vi "PH_Beckhoff_StepMot.Test.vi"() -> ()   [LabVIEW 2014, in "PH_Beckhoff_StepMot.lvlib"]
uses:
  PH_Beckhoff_StepMot.lvlib
  PH_Stepmotor_BaseClass/PH_Stepmotor_BaseClass.Axis Activity.ctl
  non_GPL/instr.lib/Beckhoff/Read and Write Data/Step Motor Klemmen/Beckhoff.Step Motor - Control Byte.ctl
  non_GPL/instr.lib/Beckhoff/Read and Write Data/Step Motor Klemmen/Beckhoff.Step Motor - Control Word.ctl
  non_GPL/instr.lib/Beckhoff/Specials/Step Motor Klemmen/Beckhoff.Step Motor - Motor Configuration.ctl
  non_GPL/instr.lib/Beckhoff/Read and Write Register/Step Motor Klemmen/Beckhoff.Step Motor - Feature Register 1.ctl
  non_GPL/instr.lib/Beckhoff/Read and Write Register/Step Motor Klemmen/Beckhoff.Step Motor - Feature Register 2.ctl
  non_GPL/instr.lib/Beckhoff/Specials/Step Motor Klemmen/Beckhoff.Step Motor - Klemmen.ctl
  non_GPL/instr.lib/Beckhoff/Read and Write Data/Step Motor Klemmen/Beckhoff.Step Motor - Status.ctl
  non_GPL/instr.lib/Beckhoff/Read and Write Data/Step Motor Klemmen/Beckhoff.Step Motor - Status Byte.ctl
  non_GPL/instr.lib/Beckhoff/Read and Write Data/Step Motor Klemmen/Beckhoff.Step Motor - Status Word.ctl
  non_GPL/instr.lib/Beckhoff/Helpers/Beckhoff Access.ctl
  non_GPL/instr.lib/Beckhoff/Helpers/Klemmendeclarer.ctl
  non_GPL/instr.lib/Beckhoff/Beckhoff - Driver np.lvlib
  PH_Common/PH_Common.lvlib
  PH_Stepmotor_BaseClass/PH_Stepmotor_BaseClass.lvlib
panel:
  in  "Go to":bool
  in  "goto pos":i32
  out "Status":T1
  out "Klemmentype":T4
  out "Position":cluster{"Target":i32, "Current":i32}
  in  "Tab Control":T5(tab)
  in  "Configuration":T6
  in  "ES enabled":bool
  in  "ES reversed":bool caption="End-Switches reversed"
  in  "Set Position":bool
  in  "Position to set":i32=10000
  in  "Register Value to set":u32 caption="Value to set"
  in  "Set Register":bool caption="Set Register Word"
  in  "Register":u32
  in  "Read Register":bool caption="Read"
  out "Register Current Value":u32 caption="Current Value"
  in  "Set Control Word":bool caption="Set Word"
  in  "Set Control Byte":bool caption="Set Byte"
  in  "Control Word":T9 caption="Word"
  in  "Control Byte":T10 caption="Byte"
  in  "Set Dig Outs":bool[](array[boolean])
  out "Current Dig Outs":bool[](array[boolean])
  out "Current Dig Ins":bool[](array[boolean])
  out "Config ready":bool
  out "Coupler found":bool
  out "Client found":bool
  out "Successfully pinged?":bool
  in  "IP":string="192.168.0.231"
  out "Error Code":string
  out "DLL Error":errorcluster
  out "Port opened?":bool
  out "Close successful":bool
  in  "Stop":bool
  out "Axis Activity":T11=enum."stopped"
  out "Loop Counter":i32
  in  "End":bool
  in  "Reset Klemme":bool
  in  "Klemme":u32=2
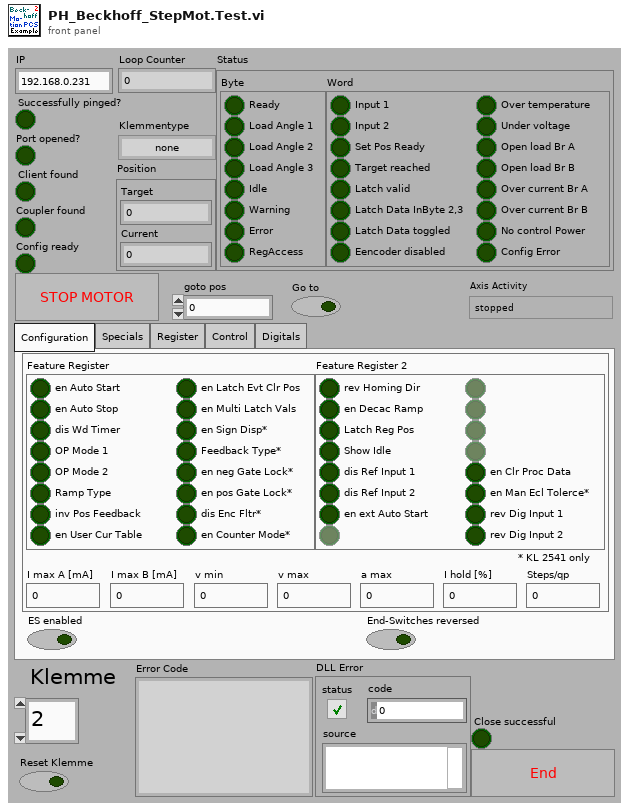
[diagram p1: front panel]
types:
  T1 = typedef "Beckhoff - Driver np.lvlib/Beckhoff.Step Motor - Status.ctl" = cluster{"Byte":T2, "Word":T3}
  T2 = typedef "Beckhoff - Driver np.lvlib/Beckhoff.Step Motor - Status Byte.ctl" = cluster{"Ready":bool, "Load Angle 1":bool, "Load Angle 2":bool, "Load Angle 3":bool, "Idle":bool, "Warning":bool, "Error":bool, "RegAccess":bool}
  T3 = typedef "Beckhoff - Driver np.lvlib/Beckhoff.Step Motor - Status Word.ctl" = cluster{"Input 1":bool, "Input 2":bool, "Set Pos Ready":bool, "Target reached":bool, "Latch valid":bool, "Latch Data InByte 2,3":bool, "Latch Data toggled":bool, "Eencoder disabled":bool, "Over temperature":bool, "Under voltage":bool, "Open load Br A":bool, "Open load Br B":bool, "Over current Br A":bool, "Over current Br B":bool, "No control Power":bool, "Config Error":bool}
  T4 = typedef "Beckhoff - Driver np.lvlib/Beckhoff.Step Motor - Klemmen.ctl" = enum16{"none", "KL 2531", "KL 2541"}
  T5 = enum32{"Configuration", "Specials", "Register", "Control", "Digitals"}
  T6 = typedef "Beckhoff - Driver np.lvlib/Beckhoff.Step Motor - Motor Configuration.ctl" = cluster{"Feature Register":T7, "I max A [mA]":dbl, "I max B [mA]":dbl, "v min":u32, "v max":u32, "a max":u32, "I hold [%]":u32, "Steps/qp":u32, "Feature Register 2":T8}
  T7 = typedef "Beckhoff - Driver np.lvlib/Beckhoff.Step Motor - Feature Register 1.ctl" = cluster{"en Auto Start":bool, "en Auto Stop":bool, "dis Wd Timer":bool, "OP Mode 1":bool, "OP Mode 2":bool, "Ramp Type":bool, "inv Pos Feedback":bool, "en User Cur Table":bool, "en Latch Evt Clr Pos":bool, "en Multi Latch Vals":bool, "en Sign Disp*":bool, "Feedback Type*":bool, "en neg Gate Lock*":bool, "en pos Gate Lock*":bool, "dis Enc Fltr*":bool, "en Counter Mode*":bool}
  T8 = typedef "Beckhoff - Driver np.lvlib/Beckhoff.Step Motor - Feature Register 2.ctl" = cluster{"rev Homing Dir":bool, "en Decac Ramp":bool, "Latch Reg Pos":bool, "Show Idle":bool, "dis Ref Input 1":bool, "dis Ref Input 2":bool, "en ext Auto Start":bool, "N/A":bool, "N/A":bool, "N/A":bool, "N/A":bool, "N/A":bool, "en Clr Proc Data":bool, "en Man Ecl Tolerce*":bool, "rev Dig Input 1":bool, "rev Dig Input 2":bool}
  T9 = typedef "Beckhoff - Driver np.lvlib/Beckhoff.Step Motor - Control Word.ctl" = cluster{"en Latch C":bool, "en Latch Input 1":bool, "en Latch Input 2":bool, "en Latch Rise Edge":bool, "en Latch Fall Edge":bool, "Get Latch Data":bool, "Toggle Latch Data":bool, "Get Position Error":bool, "Get Encoder Position":bool, "Dis mixed Decay":bool, "Set Pos":bool, "Reduced Current":bool, "Reduced Current (drivng)":bool, "Clear Position":bool, "Set Position in Process Data":bool, "N/A":bool}
  T10 = typedef "Beckhoff - Driver np.lvlib/Beckhoff.Step Motor - Control Byte.ctl" = cluster{"Enable":bool, "PLC-Stop":bool, "Start":bool, "Red Current":bool, "AutoStart":bool, "AutoStop":bool, "Reset":bool, "RegAccess":bool}
  T11 = typedef "PH_Stepmotor_BaseClass.lvlib/PH_Stepmotor_BaseClass.Axis Activity.ctl" = enum16{"No Information", "stopped", "running", "Failure", "Alarm", "stopped at backward ES", "stopped at foreward ES"}
  T12 = typedef "Beckhoff - Driver np.lvlib/Klemmendeclarer.ctl" = cluster{"Offset due to Sonderklemms":u32, "analog Inputs":u32, "analog Outputs":u32, "digital Input Bits":u32, "digital Output Bits":u32}
  T13 = typedef "Beckhoff - Driver np.lvlib/Beckhoff Access.ctl" = cluster{"DLL path":path, "AMS Net ID":cluster{"1st # of IP":u8, "2nd # of IP":u8, "3rd # of IP":u8, "4th # of IP":u8, "In Port":u8, "Out Port":u8}}
  T14 = cluster{"1st # of IP":u8, "2nd # of IP":u8, "3rd # of IP":u8, "4th # of IP":u8, u8, u8}
  T15 = enum8{"Enabled", "Disabled", "Disabled and Grayed Out"}
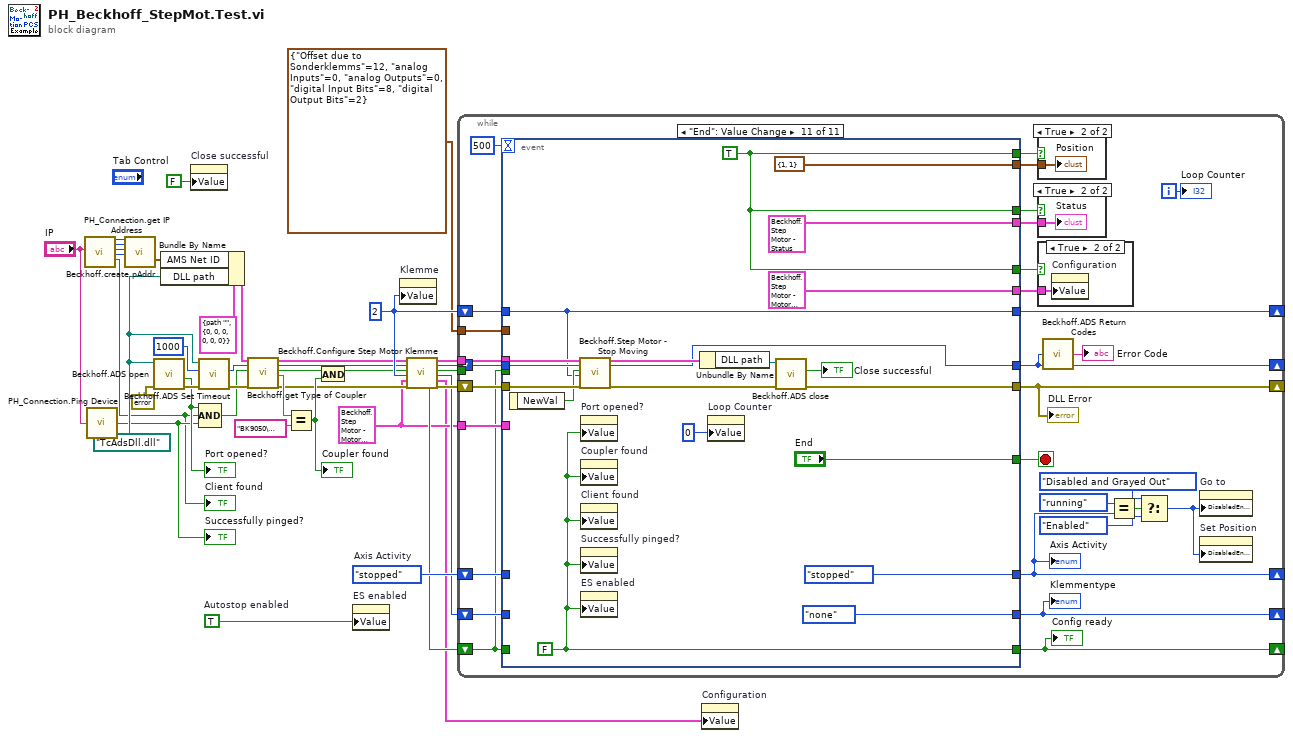
[diagram p0: block diagram]
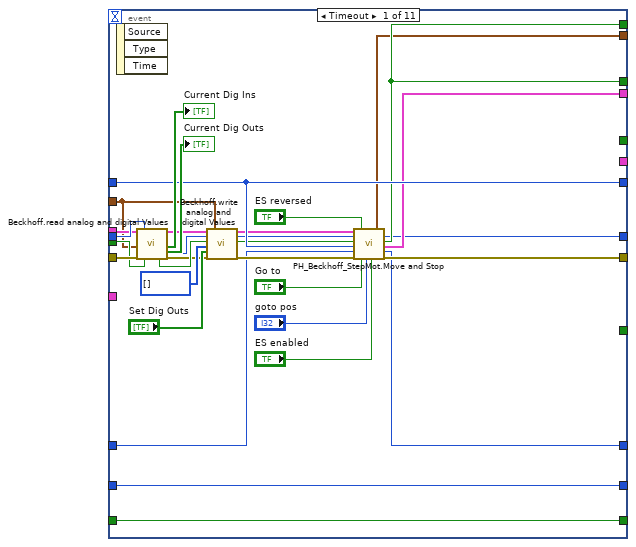
[diagram p5: hidden frame]
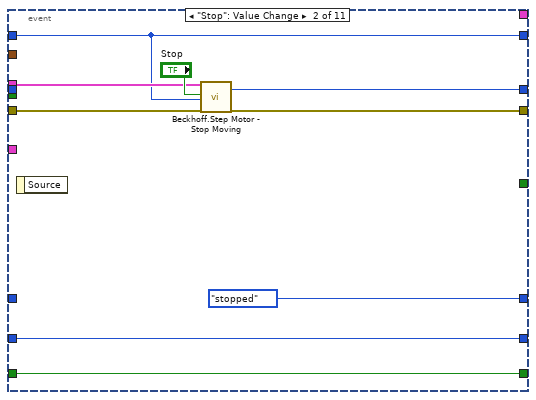
[diagram p6: hidden frame]
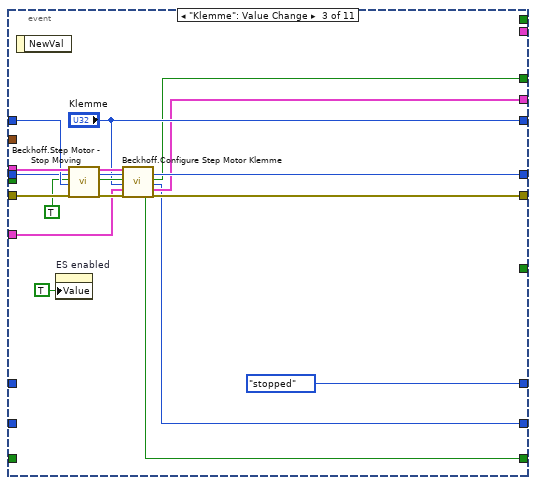
[diagram p7: hidden frame]
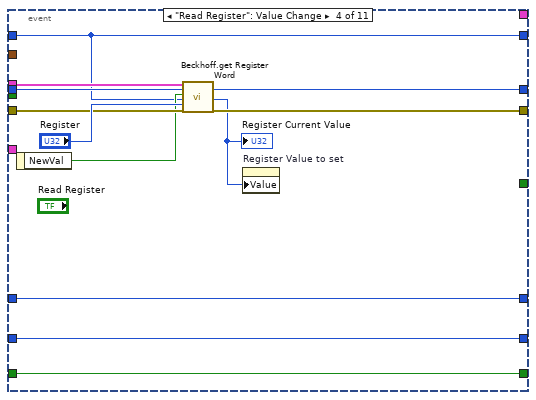
[diagram p8: hidden frame]
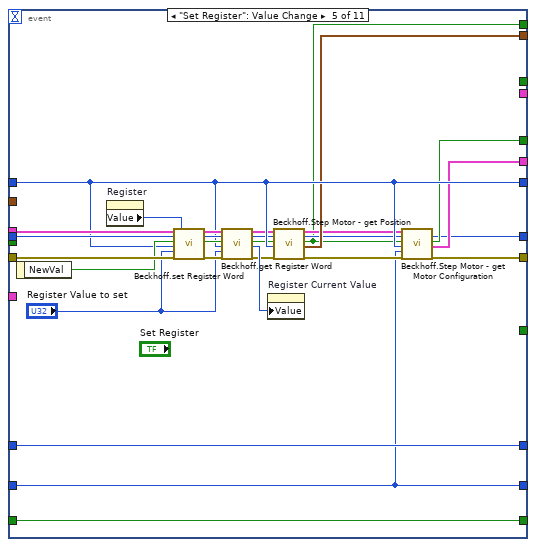
[diagram p9: hidden frame]
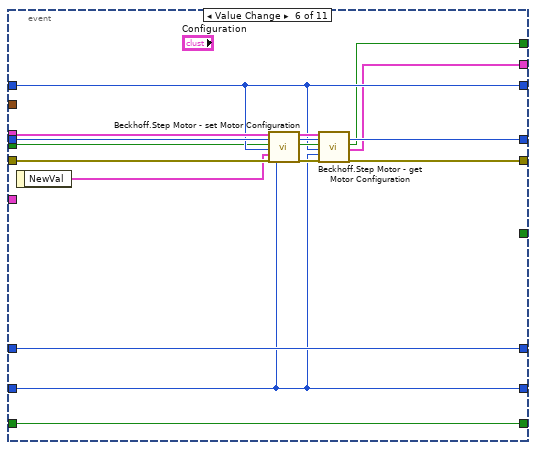
[diagram p10: hidden frame]
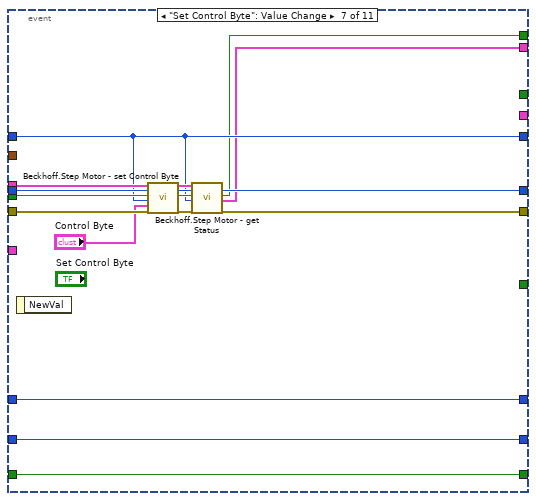
[diagram p11: hidden frame]
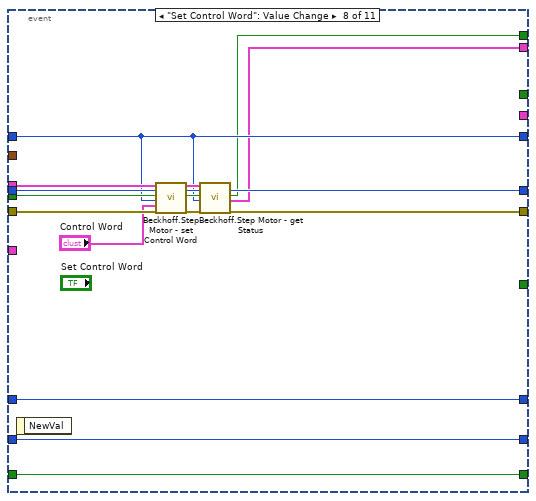
[diagram p12: hidden frame]
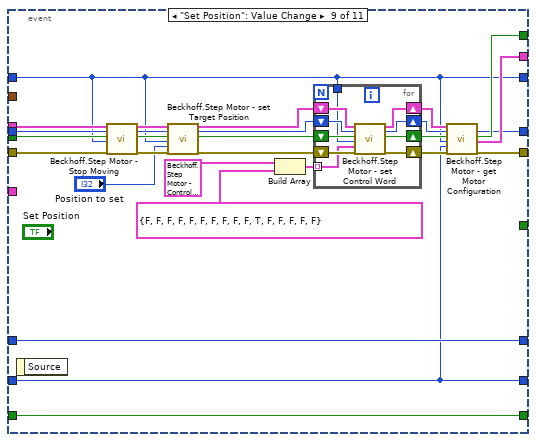
[diagram p13: hidden frame]
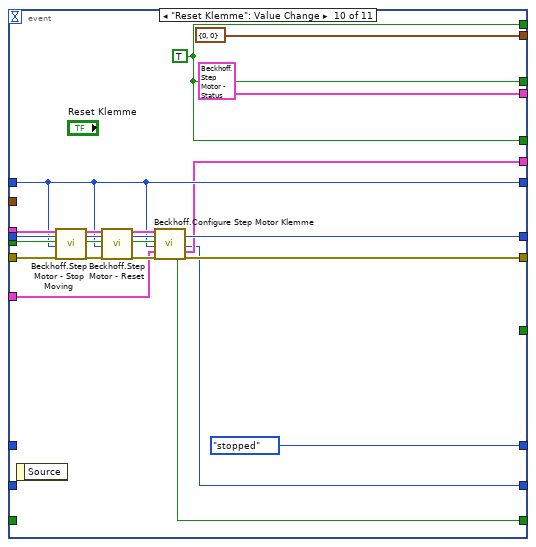
[diagram p14: hidden frame]
diagram:
  w2 = T6 {"Feature Register"={"en Auto Start"=FALSE, "en Auto Stop"=TRUE, "dis Wd Timer"=TRUE, "OP Mode 1"=TRUE, "OP Mode 2"=TRUE, "Ramp Type"=FALSE, "inv Pos Feedback"=FALSE, "en User Cur Table"=FALSE, "en Latch Evt Clr Pos"=FALSE, "en Multi Latch Vals"=FALSE, "en Sign Disp*"=FALSE, "Feedback Type*"=FALSE, "en neg Gate Lock*"=FALSE, "en pos Gate Lock*"=FALSE, "dis Enc Fltr*"=FALSE, "en Counter Mode*"=FALSE}, "I max A [mA]"=400.0, "I max B [mA]"=400.0, "v min"=10, "v max"=512, "a max"=32, "I hold [%]"=15, "Steps/qp"=4, "Feature Register 2"={"rev Homing Dir"=FALSE, "en Decac Ramp"=FALSE, "Latch Reg Pos"=FALSE, "Show Idle"=TRUE, "dis Ref Input 1"=FALSE, "dis Ref Input 2"=FALSE, "en ext Auto Start"=FALSE, "N/A"=FALSE, "N/A"=FALSE, "N/A"=FALSE, "N/A"=FALSE, "N/A"=FALSE, "en Clr Proc Data"=FALSE, "en Man Ecl Tolerce*"=FALSE, "rev Dig Input 1"=TRUE, "rev Dig Input 2"=TRUE}} ("Micos VT-80")
  w12 = u32 2 ("Klemme")
  w15 = TRUE  # Autostop enabled
  w16 = PH_Stepmotor_BaseClass.Axis_Activity."stopped"  # Axis Activity
  w31 = path "TcAdsDll.dll" ("DLL path in")
  n1 = call "PH_Connection.get IP Address.vi"("IP Name"="IP") -> ("1st # of IP"=w39:u8, "2nd # of IP"=w38:u8, "3rd # of IP"=w37:u8, "4th # of IP"=w36:u8, "Client found"=w19:bool)  [unwired: 13 in, 1 out]
  "Client found" <- w19
  n2 = call "PH_Connection.Ping Device.vi"("IP"="IP") -> ("successfully pinged?"=w25:bool)
  "Successfully pinged?" <- w25
  n3 = call "Beckhoff.create pAddr.vi"("1st # of IP"=w39, "2nd # of IP"=w38, "3rd # of IP"=w37, "4th # of IP"=w36) -> ("AMS Net ID"=w21:T14)  [unwired: 13 in, 2 out]
  n4 = call "Beckhoff.ADS open.vi"("error in"=errorcluster {"status"=FALSE, "code"=0, "source"=""}, "path in"=w31) -> ("error out"=w33:errorcluster, "Port opened?"=w26:bool)  [unwired: 3 in, 1 out]
  "Port opened?" <- w26
  n5 = Bundle By Name(cluster=T13 {"DLL path"=path "", "AMS Net ID"={"1st # of IP"=0, "2nd # of IP"=0, "3rd # of IP"=0, "4th # of IP"=0, "In Port"=0, "Out Port"=0}} ("AMS Net ID in"), "AMS Net ID"=w21, "DLL path"=w31) -> (w29:T13)
  n6 = property on="Close successful" class="Bool (strict)"("Value"=FALSE ("coupler found")) -> ()  [unwired: 2 in, 2 out]
  n7 = call "Beckhoff.ADS Set Timeout.vi"("error in"=w33, "nMs in"=u32 1000 ("nMs"), "path in"=w31) -> ("error out"=w27:errorcluster, "return type"=w28:i32)  [unwired: 6 in, 1 out]
  n8 = Compound Arithmetic op=AND(w26, w19, w25) -> (w24:bool)
  n9 = call "Beckhoff.get Type of Coupler.vi"("AMS Net ID in"=w29, "ADS Error in (0)"=w28, "Read?"=w24, "error in"=w27) -> ("AMS Net ID out"=w11:T13, "ADS Error out"=w10:i32, "Read successful?"=w17:bool, "Coupler Type"=w22:string, "error out"=w14:errorcluster)  [unwired: 11 in]
  n10 = Equal?(x=w22, y="BK9050\u0000\u0000" ("type")) -> (x = y?=w18:bool)
  "Coupler found" <- w18
  n11 = And(x=w17, y=w18) -> (x .and. y?=w9:bool)
  n12 = property on="ES enabled" class="Bool (strict)"("Value"=w15) -> ()  [unwired: 2 in, 2 out]
  n13 = property on="Klemme" class="DigNum (strict)"("Value"=w12) -> ()  [unwired: 2 in, 2 out]
  n14 = call "Beckhoff.Configure Step Motor Klemme.vi"("AMS Net ID in"=w11, "ADS Error in"=w10, "Configure?"=w9, "Klemme"=w12, "Default Configuration"=w2, "error in (no error)"=w14) -> ("Successfully configured?"=w4:bool, "AMS Net ID out"=w8:T13, "ADS Error out"=w7:i32, "Operation successful?"=w6:bool, "Klemmentype"=w5:T4, "Current Step Motor Configuration"=w1:T6, "error out"=w13:errorcluster)  [unwired: 7 in]
  n15 = while {
    shift-right: [w42] -> _
    shift-left: w16 -> [w68]
    tunnel: w8 -> [w67]
    tunnel: w6 -> [_]
    shift-right: [w61] -> _
    shift-left: w13 -> [w65]
    shift-right: [w60] -> _
    shift-left: w7 -> [w64]
    shift-right: [w57] -> _
    shift-left: w12 -> [w66]
    shift-right: [w49] -> _
    shift-left: w5 -> [w58]
    tunnel: w2 -> [w52]
    shift-right: [w48] -> _
    shift-left: w4 -> [w47]
    tunnel: T12 {"Offset due to Sonderklemms"=12, "analog Inputs"=0, "analog Outputs"=0, "digital Input Bits"=8, "digital Output Bits"=2} ("Klemmendeclarer: # of") -> [w43]
    i -> [w69]
    stop <- w62 stop-if-true
    n16 = event shown="[10] \"End\": Value Change" {
      selector: _ -> [_ _ _ _ _ _ _ _ _ _ _]
      dyn-events: _ -> [_ _ _ _ _ _ _ _ _ _ _]
      timeout: 500 -> [_ _ _ _ _ _ _ _ _ _ _]
      tunnel: w68 -> [w76 _ _ w141 w171 w188 w190 w207 w235 _ _]
      tunnel: [w86 PH_Stepmotor_BaseClass.Axis_Activity."stopped" ("Moving: 0: No; 1: forward; -1: backward") PH_Stepmotor_BaseClass.Axis_Activity."stopped" ("Moving: 0: No; 1: forward; -1: backward") w141 w171 w188 w190 w207 w235 PH_Stepmotor_BaseClass.Axis_Activity."stopped" ("Moving: 0: No; 1: forward; -1: backward") PH_Stepmotor_BaseClass.Axis_Activity."stopped" ("Moving: 0: No; 1: forward; -1: backward")] -> w42
      tunnel: w67 -> [w90 w109 w131 w139 w170 w187 w205 w222 w243 w283 w300]
      tunnel: w66 -> [w85 w107 w129 w134 w159 w177 w194 w211 w224 w268 w292]
      tunnel: w47 -> [w92 _ _ _ _ w172 w202 w219 w241 w281 _]
      tunnel: [w87 w111 w117 w143 w146 w180 w196 w214 w234 w266 w294] -> w61
      tunnel: w65 -> [w93 w108 w130 w137 w168 w185 w204 w221 w240 w280 w298]
      tunnel: [w80 w112 w125 w142 w147 w179 w195 w213 w227 w265 w293] -> w60
      tunnel: w64 -> [w91 _ w127 w138 w169 w186 w203 w220 w242 w282 w295]
      tunnel: [_ _ _ _ _ _ _ _ _ _ "End"] -> w62
      tunnel: w58 -> [w102 w106 _ w133 w145 w176 w191 w208 w225 _ _]
      tunnel: [w85 w107 "Klemme" w134 w159 w177 w194 w211 w224 w268 w292] -> w57
      tunnel: [w83 _ _ _ w150 _ _ _ _ w273 w289] -> w56
      tunnel: [w82 _ _ _ w158 _ _ _ _ cluster{"Target":i32, "Current":i32} {"Target"=0, "Current"=0} ("Position 2") cluster{"Target":i32, "Current":i32} {"Target"=1, "Current"=1} ("Position")] -> w55
      tunnel: [w83 _ _ _ _ _ w193 w209 _ w273 w289] -> w54
      tunnel: [w81 _ _ _ _ _ w192 w210 _ T1 {"Byte"={"Ready"=FALSE, "Load Angle 1"=FALSE, "Load Angle 2"=FALSE, "Load Angle 3"=FALSE, "Idle"=FALSE, "Warning"=FALSE, "Error"=FALSE, "RegAccess"=FALSE}, "Word"={"Input 1"=FALSE, "Input 2"=FALSE, "Set Pos Ready"=FALSE, "Target reached"=FALSE, "Latch valid"=FALSE, "Latch Data InByte 2,3"=FALSE, "Latch Data toggled"=FALSE, "Eencoder disabled"=FALSE, "Over temperature"=FALSE, "Under voltage"=FALSE, "Open load Br A"=FALSE, "Open load Br B"=FALSE, "Over current Br A"=FALSE, "Over current Br B"=FALSE, "No control Power"=FALSE, "Config Error"=FALSE}} ("Status") T1 {"Byte"={"Ready"=FALSE, "Load Angle 1"=FALSE, "Load Angle 2"=FALSE, "Load Angle 3"=FALSE, "Idle"=FALSE, "Warning"=FALSE, "Error"=FALSE, "RegAccess"=FALSE}, "Word"={"Input 1"=FALSE, "Input 2"=FALSE, "Set Pos Ready"=FALSE, "Target reached"=FALSE, "Latch valid"=FALSE, "Latch Data InByte 2,3"=FALSE, "Latch Data toggled"=FALSE, "Eencoder disabled"=FALSE, "Over temperature"=FALSE, "Under voltage"=FALSE, "Open load Br A"=FALSE, "Open load Br B"=FALSE, "Over current Br A"=FALSE, "Over current Br B"=FALSE, "No control Power"=FALSE, "Config Error"=FALSE}} ("Status")] -> w53
      tunnel: [_ _ w119 _ w148 w174 _ _ w228 w273 w289] -> w51
      tunnel: [_ _ w118 _ w157 w173 _ _ w229 w264 T6 {"Feature Register"={"en Auto Start"=FALSE, "en Auto Stop"=FALSE, "dis Wd Timer"=FALSE, "OP Mode 1"=FALSE, "OP Mode 2"=FALSE, "Ramp Type"=FALSE, "inv Pos Feedback"=FALSE, "en User Cur Table"=FALSE, "en Latch Evt Clr Pos"=FALSE, "en Multi Latch Vals"=FALSE, "en Sign Disp*"=FALSE, "Feedback Type*"=FALSE, "en neg Gate Lock*"=FALSE, "en pos Gate Lock*"=FALSE, "dis Enc Fltr*"=FALSE, "en Counter Mode*"=FALSE}, "I max A [mA]"=0.0, "I max B [mA]"=0.0, "v min"=0, "v max"=0, "a max"=0, "I hold [%]"=0, "Steps/qp"=0, "Feature Register 2"={"rev Homing Dir"=FALSE, "en Decac Ramp"=FALSE, "Latch Reg Pos"=FALSE, "Show Idle"=FALSE, "dis Ref Input 1"=FALSE, "dis Ref Input 2"=FALSE, "en ext Auto Start"=FALSE, "N/A"=FALSE, "N/A"=FALSE, "N/A"=FALSE, "N/A"=FALSE, "N/A"=FALSE, "en Clr Proc Data"=FALSE, "en Man Ecl Tolerce*"=FALSE, "rev Dig Input 1"=FALSE, "rev Dig Input 2"=FALSE}} ("Step Motor Configuration")] -> w50
      tunnel: [w102 w106 w115 w133 w145 w176 w191 w208 w225 w263 Beckhoff.Step_Motor_-_Klemmen."none" ("Klemmentype 2")] -> w49
      tunnel: w52 -> [_ _ w120 _ _ _ _ _ _ w267 _]
      tunnel: [w103 w105 w116 w132 w144 w175 w189 w206 w226 w262 w285] -> w48
      tunnel: w47 -> [w103 w105 _ w132 w144 w175 w189 w206 w226 _ _]
      tunnel: w43 -> [w89 _ _ _ _ _ _ _ _ _ _]
      event Timeout {
        n17 = event-data() -> ()  [unwired: 1 in, 3 out]
        n18 = call "Beckhoff.read analog and digital Values.vi"("AMS Net ID in"=w90, "Klemmendeclarer: # of"=w89, "error in"=w93, "ADS Error in (0)"=w91, "Read?"=w92) -> ("ADS Error out"=w97:i32, "read successful?"=w96:bool, "AMS Net ID out"=w94:T13, "Current Digital Inputs"=→"Current Dig Ins":bool[], "Current Digital Output"=→"Current Dig Outs":bool[], "error out"=w95:errorcluster)  [unwired: 7 in, 2 out]
        n19 = call "Beckhoff.write analog and digital Values.vi"("AMS Net ID in"=w94, "ADS Error in (0)"=w97, "Write?"=w96, "Analog Outputs to be set"=u32[] [], "Digital Outputs to be set"="Set Dig Outs", "error in"=w95, "Klemmedeclarer: # of ..."=w89) -> ("AMS Net ID out"=w84:T13, "ADS Error out"=w79:i32, "write successful?"=w78:bool, "error out"=w88:errorcluster)  [unwired: 9 in]
        n20 = call "PH_Beckhoff_StepMot.Move and Stop.vi"("AMS Net ID in"=w84, "ADS Error in"=w79, "Read and Write?"=w78, "# of Klemme [1, ...]"=w85, "Axis Activity in"=w76, "error in (no error)"=w88, "Endswitch inverted?"="ES reversed", "Move?"="Go to", "Target"="goto pos", "Endswitch?"="ES enabled") -> ("Position"=w82:cluster{"Target":i32, "Current":i32}, "ADS Error out"=w80:i32, "Read and Write succesful?"=w83:bool, "Status"=w81:T1, "Axis Activity out"=w86:T11, "error out"=w87:errorcluster)  [unwired: 3 in, 1 out]
      }
      event "Stop": Value Change {
        n21 = event-data() -> ()  [unwired: 1 in, 1 out]
        n22 = call "Beckhoff.Step Motor - Stop Moving.vi"("AMS Net ID in"=w109, "Write?"="Stop", "Klemme"=w107, "error in (no error)"=w108) -> ("ADS Error out"=w112:i32, "error out"=w111:errorcluster)  [unwired: 12 in, 2 out]
      }
      event "Klemme": Value Change {
        n23 = event-data() -> ()  [unwired: 1 in, 1 out]
        n24 = property on="ES enabled" class="Bool (strict)"("Value"=TRUE ("Autostop enabled")) -> ()  [unwired: 2 in, 2 out]
        n25 = call "Beckhoff.Step Motor - Stop Moving.vi"("AMS Net ID in"=w131, "ADS Error in (0)"=w127, "Write?"=TRUE, "Klemme"=w129, "error in (no error)"=w130) -> ("AMS Net ID out"=w126:T13, "ADS Error out"=w124:i32, "Write successful?"=w123:bool, "error out"=w122:errorcluster)  [unwired: 11 in]
        n26 = call "Beckhoff.Configure Step Motor Klemme.vi"("AMS Net ID in"=w126, "ADS Error in"=w124, "Configure?"=w123, "Klemme"="Klemme", "Default Configuration"=w120, "error in (no error)"=w122) -> ("Successfully configured?"=w116:bool, "ADS Error out"=w125:i32, "Operation successful?"=w119:bool, "Klemmentype"=w115:T4, "Current Step Motor Configuration"=w118:T6, "error out"=w117:errorcluster)  [unwired: 7 in, 1 out]
      }
      event "Read Register": Value Change {
        n27 = event-data() -> ("NewVal"=w136:bool)  [unwired: 1 in]
        n28 = call "Beckhoff.get Register Word.vi"("AMS Net ID in"=w139, "ADS Error in (0)"=w138, "Read?"=w136, "# of Klemme [1 ...]"=w134, "Register"="Register", "error in"=w137) -> ("ADS Error out"=w142:i32, "Current value"=w135:u32, "error out"=w143:errorcluster)  [unwired: 9 in, 2 out]
        "Register Current Value" <- w135
        n29 = property on="Register Value to set" class="DigNum (strict)"("Value"=w135) -> ()  [unwired: 2 in, 2 out]
      }
      event "Set Register": Value Change {
        n30 = event-data() -> ("NewVal"=w167:bool)  [unwired: 1 in]
        n31 = property on="Register" class="DigNum (strict)"() -> ("Value"=w166:u32)  [unwired: 2 in, 2 out]
        n32 = call "Beckhoff.set Register Word.vi"("AMS Net ID in"=w170, "ADS Error in (0)"=w169, "Write?"=w167, "# of Klemme [1 ...]"=w159, "Value to set"="Register Value to set", "error in"=w168, "Register"=w166) -> ("AMS Net ID out"=w165:T13, "ADS Error out"=w162:i32, "Write successful?"=w163:bool, "error out"=w164:errorcluster)  [unwired: 9 in]
        n33 = call "Beckhoff.get Register Word.vi"("AMS Net ID in"=w165, "ADS Error in (0)"=w162, "Read?"=w163, "# of Klemme [1 ...]"=w159, "Register"="Register Value to set", "error in"=w164) -> ("AMS Net ID out"=w156:T13, "ADS Error out"=w155:i32, "Read successful?"=w154:bool, "Current value"=w161:u32, "error out"=w153:errorcluster)  [unwired: 9 in]
        n34 = property on="Register Current Value" class="DigNum (strict)"("Value"=w161) -> ()  [unwired: 2 in, 2 out]
        n35 = call "Beckhoff.Step Motor - get Position.vi"("AMS Net ID in"=w156, "ADS Error in (0)"=w155, "Read?"=w154, "# of Klemme [1, ...]"=w159, "error in (no error)"=w153) -> ("AMS Net ID out"=w152:T13, "ADS Error out"=w151:i32, "Read successful?"=w150:bool, "Position"=w158:cluster{"Target":i32, "Current":i32}, "error out"=w149:errorcluster)  [unwired: 10 in]
        n36 = call "Beckhoff.Step Motor - get Motor Configuration.vi"("AMS Net ID in"=w152, "ADS Error in"=w151, "Read?"=w150, "# of Klemme [1 ...]"=w159, "Klemmentype"=w145, "error in (no error)"=w149) -> ("ADS Error out"=w147:i32, "Operation successful?"=w148:bool, "current Step Motor Configuration"=w157:T6, "error out"=w146:errorcluster)  [unwired: 9 in, 1 out]
      }
      event Value Change {
        n37 = event-data() -> ("NewVal"=w178:T6)  [unwired: 1 in]
        n38 = call "Beckhoff.Step Motor - set Motor Configuration.vi"("AMS Net ID in"=w187, "ADS Error in"=w186, "Write?"=w172, "# of Klemme [1 ...]"=w177, "Step Motor Configuration to set"=w178, "error in (no error)"=w185, "Klemmentyp"=w176) -> ("AMS Net ID out"=w184:T13, "ADS Error out"=w183:i32, "Operation successful?"=w182:bool, "error out"=w181:errorcluster)  [unwired: 9 in]
        n39 = call "Beckhoff.Step Motor - get Motor Configuration.vi"("AMS Net ID in"=w184, "ADS Error in"=w183, "Read?"=w182, "# of Klemme [1 ...]"=w177, "Klemmentype"=w176, "error in (no error)"=w181) -> ("ADS Error out"=w179:i32, "Operation successful?"=w174:bool, "current Step Motor Configuration"=w173:T6, "error out"=w180:errorcluster)  [unwired: 9 in, 1 out]
      }
      event "Set Control Byte": Value Change {
        n40 = event-data() -> ()  [unwired: 1 in, 1 out]
        n41 = call "Beckhoff.Step Motor - set Control Byte.vi"("AMS Net ID in"=w205, "ADS Error in (0)"=w203, "Write?"=w202, "# of Klemme [1, ...]"=w194, "Control Byte"="Control Byte", "error in (no error)"=w204) -> ("AMS Net ID out"=w200:T13, "ADS Error out"=w198:i32, "Write successful?"=w197:bool, "error out"=w199:errorcluster)  [unwired: 10 in]
        n42 = call "Beckhoff.Step Motor - get Status.vi"("AMS Net ID in"=w200, "ADS Error in (0)"=w198, "Read?"=w197, "# of Klemme [1, ...]"=w194, "error in (no error)"=w199) -> ("ADS Error out"=w195:i32, "Read successful?"=w193:bool, "Status"=w192:T1, "error out"=w196:errorcluster)  [unwired: 10 in, 1 out]
      }
      event "Set Control Word": Value Change {
        n43 = event-data() -> ()  [unwired: 1 in, 1 out]
        n44 = call "Beckhoff.Step Motor - set Control Word.vi"("AMS Net ID in"=w222, "ADS Error in (0)"=w220, "Write?"=w219, "# of Klemme [1, ...]"=w211, "Control Word"="Control Word", "error in (no error)"=w221) -> ("AMS Net ID out"=w218:T13, "ADS Error out"=w216:i32, "Write successful?"=w215:bool, "error out"=w217:errorcluster)  [unwired: 10 in]
        n45 = call "Beckhoff.Step Motor - get Status.vi"("AMS Net ID in"=w218, "ADS Error in (0)"=w216, "Read?"=w215, "# of Klemme [1, ...]"=w211, "error in (no error)"=w217) -> ("ADS Error out"=w213:i32, "Read successful?"=w209:bool, "Status"=w210:T1, "error out"=w214:errorcluster)  [unwired: 10 in, 1 out]
      }
      event "Set Position": Value Change {
        n46 = event-data() -> ()  [unwired: 1 in, 1 out]
        n47 = call "Beckhoff.Step Motor - Stop Moving.vi"("AMS Net ID in"=w243, "ADS Error in (0)"=w242, "Write?"=w241, "Klemme"=w224, "error in (no error)"=w240) -> ("AMS Net ID out"=w239:T13, "ADS Error out"=w238:i32, "Write successful?"=w237:bool, "error out"=w236:errorcluster)  [unwired: 11 in]
        n48 = call "Beckhoff.Step Motor - set Target Position.vi"("AMS Net ID in"=w239, "ADS Error in (0)"=w238, "Write?"=w237, "# of Klemme [1, ...]"=w224, "Target Position"="Position to set", "error in (no error)"=w236) -> ("AMS Net ID out"=w232:T13, "ADS Error out"=w248:i32, "Write successful?"=w247:bool, "error out"=w250:errorcluster)  [unwired: 10 in]
        n49 = Build Array(T9 {"en Latch C"=FALSE, "en Latch Input 1"=FALSE, "en Latch Input 2"=FALSE, "en Latch Rise Edge"=FALSE, "en Latch Fall Edge"=FALSE, "Get Latch Data"=FALSE, "Toggle Latch Data"=FALSE, "Get Position Error"=FALSE, "Get Encoder Position"=FALSE, "Dis mixed Decay"=FALSE, "Set Pos"=FALSE, "Reduced Current"=FALSE, "Reduced Current (drivng)"=FALSE, "Clear Position"=FALSE, "Set Position in Process Data"=FALSE, "N/A"=FALSE} ("Control Word"), T9 {"en Latch C"=FALSE, "en Latch Input 1"=FALSE, "en Latch Input 2"=FALSE, "en Latch Rise Edge"=FALSE, "en Latch Fall Edge"=FALSE, "Get Latch Data"=FALSE, "Toggle Latch Data"=FALSE, "Get Position Error"=FALSE, "Get Encoder Position"=FALSE, "Dis mixed Decay"=FALSE, "Set Pos"=TRUE, "Reduced Current"=FALSE, "Reduced Current (drivng)"=FALSE, "Clear Position"=FALSE, "Set Position in Process Data"=FALSE, "N/A"=FALSE} ("Control Word")) -> (w245:T9[])
        n50 = for {
          tunnel: w245 -> [w254] mode=indexing
          shift-right: [w259] -> w249
          shift-left: w250 -> [w260]
          shift-right: [w255] -> w233
          shift-left: w248 -> [w257]
          tunnel: w224 -> [w253]
          shift-right: [w252] -> w231
          shift-left: w232 -> [w258]
          shift-right: [w251] -> w230
          shift-left: w247 -> [w256]
          n51 = call "Beckhoff.Step Motor - set Control Word.vi"("AMS Net ID in"=w258, "ADS Error in (0)"=w257, "Write?"=w256, "# of Klemme [1, ...]"=w253, "Control Word"=w254, "error in (no error)"=w260) -> ("AMS Net ID out"=w252:T13, "ADS Error out"=w255:i32, "Write successful?"=w251:bool, "error out"=w259:errorcluster)  [unwired: 10 in]
        }
        n52 = call "Beckhoff.Step Motor - get Motor Configuration.vi"("AMS Net ID in"=w231, "ADS Error in"=w233, "Read?"=w230, "# of Klemme [1 ...]"=w224, "Klemmentype"=w225, "error in (no error)"=w249) -> ("ADS Error out"=w227:i32, "Operation successful?"=w228:bool, "current Step Motor Configuration"=w229:T6, "error out"=w234:errorcluster)  [unwired: 9 in, 1 out]
      }
      event "Reset Klemme": Value Change {
        w273 = TRUE ("Read successful?")
        n53 = event-data() -> ()  [unwired: 1 in, 1 out]
        n54 = call "Beckhoff.Step Motor - Stop Moving.vi"("AMS Net ID in"=w283, "ADS Error in (0)"=w282, "Write?"=w281, "Klemme"=w268, "error in (no error)"=w280) -> ("AMS Net ID out"=w279:T13, "ADS Error out"=w277:i32, "Write successful?"=w276:bool, "error out"=w278:errorcluster)  [unwired: 11 in]
        n55 = call "Beckhoff.Step Motor - Reset.vi"("AMS Net ID in"=w279, "ADS Error in (0)"=w277, "Write?"=w276, "Klemme"=w268, "error in (no error)"=w278) -> ("AMS Net ID out"=w271:T13, "ADS Error out"=w269:i32, "Write successful?"=w270:bool, "error out"=w272:errorcluster)  [unwired: 11 in]
        n56 = call "Beckhoff.Configure Step Motor Klemme.vi"("AMS Net ID in"=w271, "ADS Error in"=w269, "Configure?"=w270, "Klemme"=w268, "Default Configuration"=w267, "error in (no error)"=w272) -> ("Successfully configured?"=w262:bool, "ADS Error out"=w265:i32, "Klemmentype"=w263:T4, "Current Step Motor Configuration"=w264:T6, "error out"=w266:errorcluster)  [unwired: 7 in, 2 out]
      }
      event "End": Value Change {
        w289 = TRUE ("Read successful?")
        w285 = FALSE ("Port opened?")
        n57 = event-data() -> ("NewVal"=w296:bool)  [unwired: 1 in]
        n58 = call "Beckhoff.Step Motor - Stop Moving.vi"("AMS Net ID in"=w300, "ADS Error in (0)"=w295, "Write?"=w296, "Klemme"=w292, "error in (no error)"=w298) -> ("AMS Net ID out"=w299:T13, "ADS Error out"=w293:i32, "error out"=w297:errorcluster)  [unwired: 11 in, 1 out]
        n59 = property on="Port opened?" class="Bool (strict)"("Value"=w285) -> ()  [unwired: 2 in, 2 out]
        n60 = property on="Coupler found" class="Bool (strict)"("Value"=w285) -> ()  [unwired: 2 in, 2 out]
        n61 = property on="Client found" class="Bool (strict)"("Value"=w285) -> ()  [unwired: 2 in, 2 out]
        n62 = property on="Successfully pinged?" class="Bool (strict)"("Value"=w285) -> ()  [unwired: 2 in, 2 out]
        n63 = property on="ES enabled" class="Bool (strict)"("Value"=w285) -> ()  [unwired: 2 in, 2 out]
        n64 = Unbundle By Name(w299) -> ("DLL path"=w301:path)
        n65 = property on="Loop Counter" class="DigNum (strict)"("Value"=0 ("Loop Counter")) -> ()  [unwired: 2 in, 2 out]
        n66 = call "Beckhoff.ADS close.vi"("error in"=w297, "path in"=w301) -> ("error out"=w294:errorcluster, "Close sucessful"=→"Close successful":bool)  [unwired: 4 in]
      }
    }
    "DLL Error" <- w61
    "Axis Activity" <- w42
    "Klemmentype" <- w49
    "Config ready" <- w48
    n67 = case shown="True" w56 {
      tunnel: w55 -> [_ w72]
      frame False {
      }
      frame True {
        "Position" <- w72
      }
    }
    n68 = case shown="True" w54 {
      tunnel: w53 -> [_ w71]
      frame False {
      }
      frame True {
        "Status" <- w71
      }
    }
    n69 = case shown="True" w51 {
      tunnel: w50 -> [_ w70]
      frame False {
      }
      frame True {
        n70 = property on="Configuration" class="Clust (strict)"("Value"=w70) -> ()  [unwired: 2 in, 2 out]
      }
    }
    n71 = call "Beckhoff.ADS Return Codes.vi"("ADS Error"=w60) -> ("Error Code"=→"Error Code":string)
    n72 = Equal?(x=PH_Stepmotor_BaseClass.Axis_Activity."running", y=w42) -> (x = y?=w40:bool)
    n73 = Select(t=T15."Disabled and Grayed Out" ("Disabled"), s=w40, f=T15."Enabled" ("Disabled")) -> (s? t:f=w44:T15)
    n74 = property on="Go to" class="Bool"("DisabledEnum"=w44) -> ()  [unwired: 2 in, 2 out]
    n75 = property on="Set Position" class="Bool"("DisabledEnum"=w44) -> ()  [unwired: 2 in, 2 out]
    "Loop Counter" <- w69
  }
  n76 = property on="Configuration" class="Clust (strict)"("Value"=w1) -> ()  [unwired: 2 in, 2 out]
